vi "Shooter.vi"(11 "State Control":enum16{"Open", "Run", "End"}(ring)) -> ()   [LabVIEW 2013]
uses:
  <vilib>/Rock Robotics/SystemInterfaces/DIO/FPGA_DIOPWMChannel.ctl
  <vilib>/Rock Robotics/WPI/MotorControl/WPI_MotorControlOpen Talon.vi
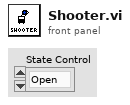
[diagram p1: front panel]
types:
  T1 = typedef "FPGA_DIOPWMChannel.ctl" = enum8{"PWM 1", "PWM 2", "PWM 3", "PWM 4", "PWM 5", "PWM 6", "PWM 7", "PWM 8", "PWM 9", "PWM 10", "Invalid"}
  T2 = typedef "WPI_MotorControlDeviceRef.ctl" = cluster{"DeviceStatus":errorcluster, "Type":enum16{"PWM", "CAN"}, "PWM":cluster{"Digital Module":T3, "PWM Channel":T1, "DeadBand":T4}, "CAN":cluster{"Device Number":u8, "Control Mode":T5, "Semaphore":T6, "Max Vout":dbl}, "Invert":bool, "TransformRef":T7, "InvTransformRef":T7}
  T3 = typedef "FPGA_TypedefDigitalModule.ctl" = enum16{"Digital Module 1", "Digital Module 2"}
  T4 = typedef "WPI_PWMDeadband.ctl" = cluster{"Name":string, "maxPositivePwm":i32, "minPositivePwm":i32, "centerPwm":i32, "maxNegativePwm":i32, "minNegativePwm":i32, "angularRange":u16}
  T5 = typedef "WPI_CANJaguar_ControlMode.ctl" = enum8{"Percent VBus", "Current", "Speed", "Position", "Voltage"}
  T6 = typedef "Semaphore RefNum" = refnum<k1>
  T7 = typedef "WPI_PWMTransform_ConPane.ctl" = refnum<vi>
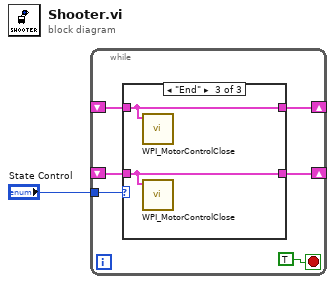
[diagram p0: block diagram]
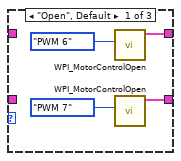
[diagram p2: hidden frame]
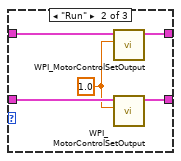
[diagram p3: hidden frame]
diagram:
  n1 = while {
    shift-right: [w7] -> _
    shift-left: _ -> [w6]
    tunnel: "State Control" -> [w5]
    shift-right: [w3] -> _
    shift-left: _ -> [w2]
    stop <- TRUE stop-if-true
    n2 = case shown="\"End\"" w5 {
      tunnel: [w9 w13 w18] -> w7
      tunnel: w6 -> [_ w15 w18]
      tunnel: [w8 w12 w17] -> w3
      tunnel: w2 -> [_ w16 w17]
      frame "Open", Default {
        n3 = call-poly <vilib>:"WPI_MotorControlOpen.vi"("PWM Channel"=FPGA_DIOPWMChannel."PWM 6" ("PWMChannel")) -> ("MotorControlDeviceRef"=w9:T2)  [unwired: 9 in, 1 out]
        n4 = call-poly <vilib>:"WPI_MotorControlOpen.vi"("PWM Channel"=FPGA_DIOPWMChannel."PWM 7" ("PWMChannel")) -> ("MotorControlDeviceRef"=w8:T2)  [unwired: 9 in, 1 out]
      }
      frame "Run" {
        w14 = 1.0 ("Output")
        n5 = call <vilib>:"WPI_MotorControlSetOutput.vi"("Output"=w14, "MotorControlDevRef"=w15) -> ("MotorControlDevRef"=w13:T2)  [unwired: 7 in, 2 out]
        n6 = call <vilib>:"WPI_MotorControlSetOutput.vi"("Output"=w14, "MotorControlDevRef"=w16) -> ("MotorControlDevRef"=w12:T2)  [unwired: 7 in, 2 out]
      }
      frame "End" {
        n7 = call <vilib>:"WPI_MotorControlClose.vi"("MotorControlDevRef"=w18) -> ()  [unwired: 10 in, 1 out]
        n8 = call <vilib>:"WPI_MotorControlClose.vi"("MotorControlDevRef"=w17) -> ()  [unwired: 10 in, 1 out]
      }
    }
  }
